vi "AH Bridge Setup Original.vi"(3 "AH 2500?":bool, 4 "AVE TIME":u32, 5 "Return Dissapation":u8, 6 "Instrument Address":refnum<visa-resource-name>) -> (0 "error out":errorcluster, 2 "dup VISA session":refnum<visa-resource-name>)   [LabVIEW 2025]
doc: "Author: Scott Hannahs <sth@magnet.fsu.edu>\n\nThis software is licensed for use under the “MIT License\"\nCopyright (c) 2025 Scott Hannahs, sth@sth@magnet.sthnet.net\n\nPermission is hereby granted, free of charge, to any person obtaining a copy of this software and associated documentation files (the \"Software\"), to deal in the Software without restriction, including without limitation the rights to use, copy, modify, merge, publish, distribute, sublicense, and/or sell copies of the Software, and to permit persons to whom the Software is furnished to do so, subject to the following conditions: The above copyright notice and this permission notice shall be included in all copies or substantial portions of the Software.\n\nTHE SOFTWARE IS PROVIDED \"AS IS\", WITHOUT WARRANTY OF ANY KIND, EXPRESS OR IMPLIED, INCLUDING BUT NOT LIMITED TO THE WARRANTIES OF MERCHANTABILITY, FITNESS FOR A PARTICULAR PURPOSE AND NONINFRINGEMENT. IN NO EVENT SHALL THE AUTHORS OR COPYRIGHT HOLDERS BE LIABLE FOR ANY CLAIM, DAMAGES OR OTHER LIABILITY, WHETHER IN AN ACTION OF CONTRACT, TORT OR OTHERWISE, ARISING FROM, OUT OF OR IN CONNECTION WITH THE SOFTWARE OR THE USE OR OTHER DEALINGS IN THE SOFTWARE."
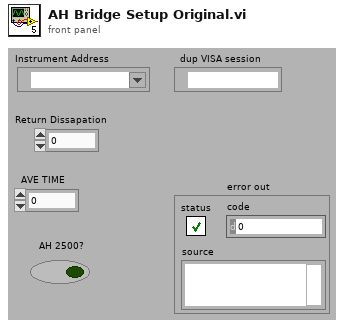
[diagram p1: front panel]
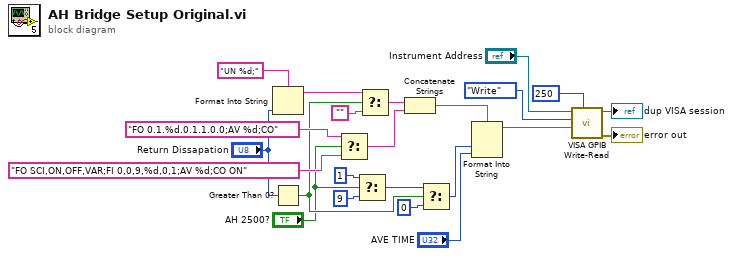
[diagram p0: block diagram]
diagram:
  n1 = Format Into String(format string="UN %d;" ("Input String"), "Return Dissapation") -> (resulting string=w19:string)  [unwired: 2 in, 1 out]
  n2 = Greater Than 0?(x="Return Dissapation") -> (x > 0?=w5:bool)
  n3 = Select(t="FO 0.1.%d.0.1.1.0.0;AV %d;CO", s="AH 2500?", f="FO SCI,ON,OFF,VAR;FI 0,0,9,%d,0,1;AV %d;CO ON") -> (s? t:f=w12:string)
  n4 = Select(t=1, s="AH 2500?", f=9 ("t")) -> (s? t:f=w9:i32)
  n5 = Select(t=w19, s=w5, f="") -> (s? t:f=w21:string)
  n6 = Concatenate Strings(w21, w12) -> (w17:string)
  n7 = Select(t=w9, s=w5, f=0) -> (s? t:f=w16:i32)
  n8 = Format Into String(format string=w17, w16, "AVE TIME") -> (resulting string=w22:string)  [unwired: 2 in, 1 out]
  n9 = call "VISA GPIB Write-Read.vi"("Wait (ms)"=u32 250 ("wait (mS)"), "Command"=w22, "Action"=enum16{"Write", "Read", "Write & Read"}."Write", "VISA resource name"="Instrument Address") -> ("error out"=→"error out":errorcluster, "dup VISA Session"=→"dup VISA session":refnum<visa-resource-name>)  [unwired: 4 in, 2 out]
